vi "Check ID Valid.vi"(8 "error in (no error)":errorcluster caption="错误输入（无错误）", 9 "Label":T1=44 format="0x%02x" items=["Image Seperator"=44, "Extension Introducer"=33, "Graphic Control Label"=249, "Comment Label"=254, "PlainText Label"=1, "Gif Trailor"=59, "Application Label"=255], 10 "ID":T1=44 format="0x%02x" items=["Image Seperator"=44, "Extension Introducer"=33, "Graphic Control Label"=249, "Comment Label"=254, "PlainText Label"=1, "Gif Trailor"=59, "Application Label"=255], 11 "Gif Image 输入":refnum<class "Gif Image.lvclass"> caption="DNL_LabVIEW Object in") -> (0 "error out":errorcluster caption="错误输出", 1 "Label Valid":bool, 2 "ID Valid":bool, 3 "Gif Image 输出":refnum<class "Gif Image.lvclass"> caption="DNL_LabVIEW Object out")   [LabVIEW 2011, in "Gif Image.lvclass"]
uses:
  Gif Image.lvclass
  Control/ID Charactor.ctl
  Gif Image.lvclass/Gif Image.ctl
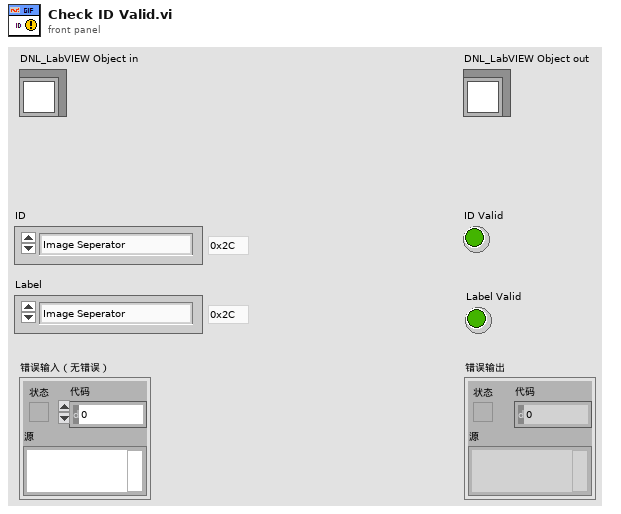
[diagram p1: front panel]
types:
  T1 = typedef "Gif Image.lvclass/ID Charactor.ctl" = u8
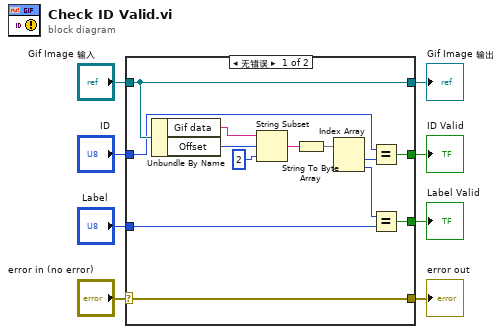
[diagram p0: block diagram]
diagram:
  n1 = case shown="无错误" "error in (no error)" {
    selector: "error in (no error)" -> [w21 w23]
    tunnel: [w21 w23] -> w7
    tunnel: [w17 w22] -> w5
    tunnel: "Gif Image 输入" -> [w17 w22]
    tunnel: [w16 _] -> w4
    tunnel: "ID" -> [w15 _]
    tunnel: "Label" -> [w11 _]
    tunnel: [w9 _] -> w1
    frame No Error {
      n2 = Unbundle By Name(w17) -> ("Gif data"=w20:string, "Offset"=w19:i32)
      n3 = String Subset(string=w20, offset (0)=w19, length (rest)=2 ("长度（剩余）")) -> (substring=w14:string)
      n4 = String To Byte Array(string=w14) -> (unsigned byte array=w13:u8[])
      n5 = Index Array(array=w13) -> (element #1=w12:u8, element #2=w10:u8)  [unwired: 2 in]
      n6 = Equal?(x=w15, y=w12) -> (x = y?=w16:bool)
      n7 = Equal?(x=w10, y=w11) -> (x = y?=w9:bool)
    }
    frame Error {
    }
  }
  "error out" <- w7
  "Gif Image 输出" <- w5
  "ID Valid" <- w4
  "Label Valid" <- w1
